vi "Global Quit Event Holder.vi"() -> ()   [LabVIEW 2014, in "LQ Core.lvlib" / "LQCoreEngine.lvclass"]
uses:
  LQCoreEngine.lvclass
panel:
  in  "Quit Event":refnum<user-event>
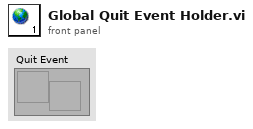
[diagram p1: front panel]
diagram:
